vi "Error Code Dialog.vi"(8 "error in":errorcluster, 10 "Library":refnum<class "Library.lvclass">, 11 "Project":refnum<class "Project.lvclass">) -> (0 "error out":errorcluster, 1 "Cancel Out":bool, 2 "Error Name":string, 3 "Project out":refnum<class "Project.lvclass">, 5 "Error VI Tag":string)   [LabVIEW 2020, in "Panther Dashboard.lvlib"]
uses:
  Panther Dashboard.lvlib
  Controls/Continue.ctl
  Controls/Cancel.ctl
  Controls/MulticolumListbox.ctl
  Class/Library/Library.lvclass
  C:/GitClones/PantherDashboard/src/LabVIEW/Panther Dashboard/Class/LabVIEWItem/LabVIEWItem.lvclass
  Class/Project/Project.lvclass
  Class/Project/Project.lvclass/Project.ctl
  Class/Library/Library.lvclass/Library.ctl
  Class/LabVIEWItem/LabVIEWItem.lvclass/LabVIEWItem.ctl
  Class/LabVIEWItem/Item Type--enum.ctl
  Class/LabVIEWItem/Read Item Tag.vi
  Class/Project/Read Project Ref.vi
  Class/Project/Read Main App Inst Ref.vi
  Class/Library/Read Library Ref.vi
  Class/Library/Read Type.vi
  Class/VI/VI.lvclass
  Class/LabVIEWItem/LabVIEWItem.lvclass
panel:
  in  "Error Description":string
  in  "Current Error VIs Values":T1
  in  "Error Name (do not add --error.vi)":string
  in  "Continue":T2
  in  "Cancel":T3
  in  "Error Code":i32
  # "These are the benefits of having Error Constant VIs\n\n1. Centralized Error Management:\n   - Single Point of Editing: by storing error codes and descriptions in constants, you can modify them in one place, ensuring consistency across the entire application. This streamlines maintenance and avoids potential errors due to inconsistencies.\n   - Enhanced Organization: Grouping error-related information in constants improves code readability and understanding. It also makes it easier to quickly locate and update error-related logic.\n\n2. Improved Code Readability:\n   - Clearer Meaning: Instead of using raw error codes directly in code, constants provide meaningful names for errors, making code more self-explanatory and easier for others to comprehend.\n   - Reduced Redundancy: Constants eliminate the need to repeatedly define error codes and descriptions throughout the code, reducing redundancy and improving code maintainability.\n\n3. Error Tracking and Debugging:\n   - Identifying Error Sources: By using constant VIs, you can easily track where specific errors are being generated within the application. This aids in debugging and pinpointing the root causes of issues.\n   - Debugging Efficiency: Constants make it easier to search for error-related code and analyze error handling logic, facilitating debugging and problem resolution.\n\n4. Flexibility for Customization:\n   - Adaptability: If error codes or descriptions need to change, you can easily update them in the constant VIs without having to modify code in multiple locations. This allows for quick adjustments and customization as needed.\n\nRanges of Custom Error Codes defined by NI:\n     –8999  through –8000\n       5000  through   9999\n  500,000  through 599,999"
  # "TIP: Doble click to open --error.vi Block Diagram"
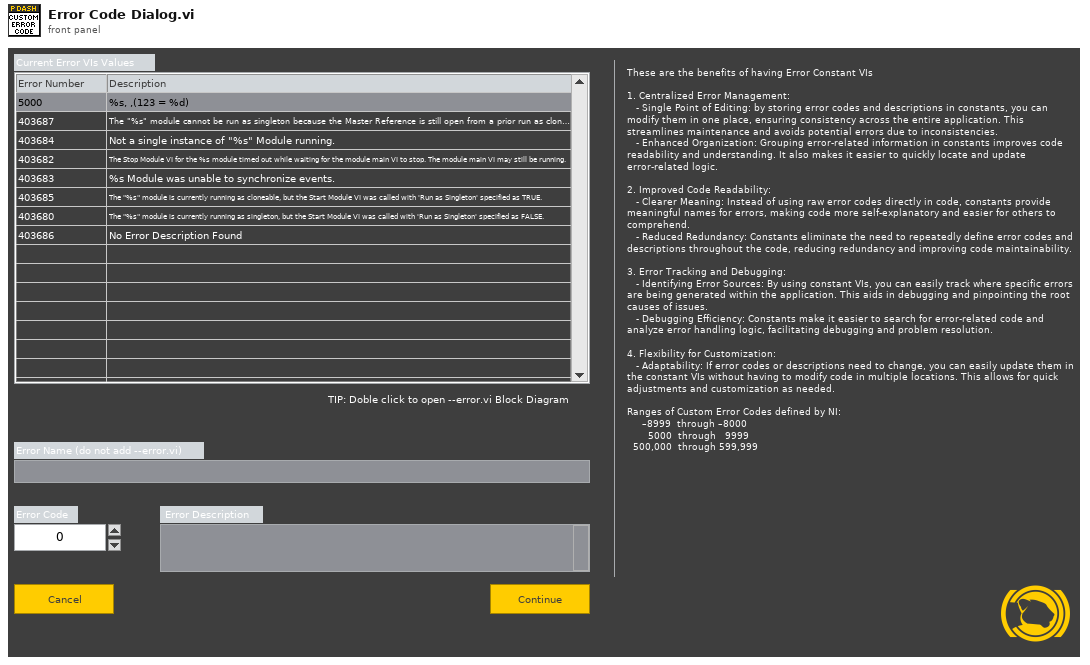
[diagram p1: front panel]
types:
  T1 = typedef "MulticolumListbox.ctl" = i32
  T2 = typedef "Continue.ctl" = bool
  T3 = typedef "Cancel.ctl" = bool
  T4 = typedef "Panther Dashboard.lvlib/Module type--enum.ctl" = enum16{"Singleton", "Cloneable"}
  T5 = typedef "Panther Dashboard.lvlib/LabVIEWItem.lvclass/Item Type--enum.ctl" = enum16{"Requests", "Broadcasts", "Request and Wait for Reply", "Round Trip", "» Public API VIs", "» Constant VIs", "» Error VIs", "Module", "Project", "No Drag Selection"}
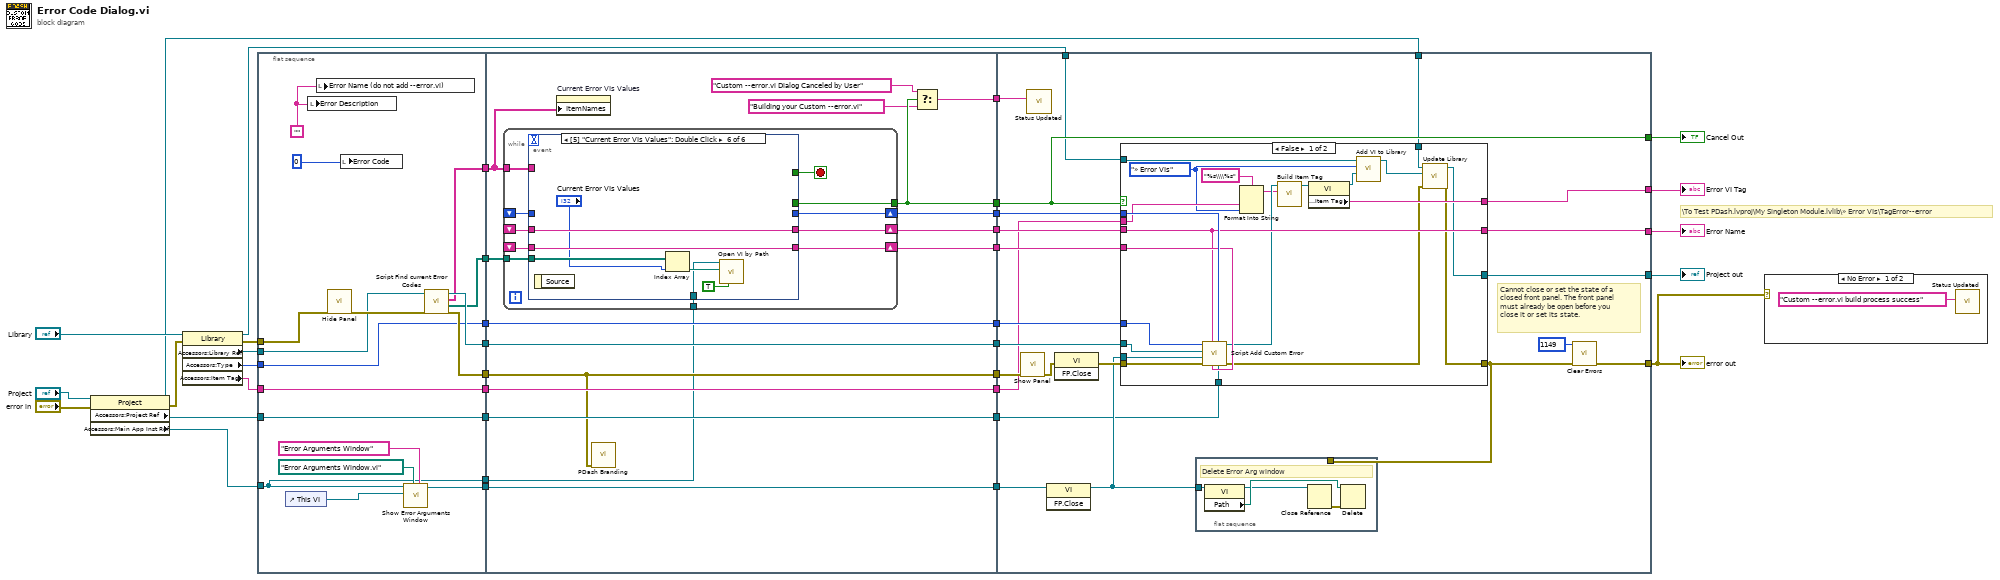
[diagram p0: block diagram]
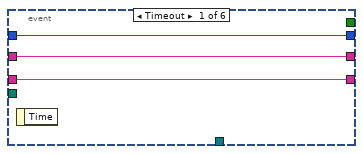
[diagram p3: hidden frame]
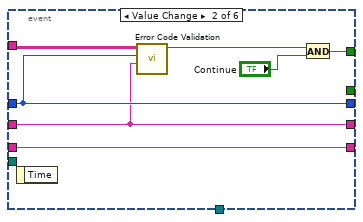
[diagram p4: hidden frame]
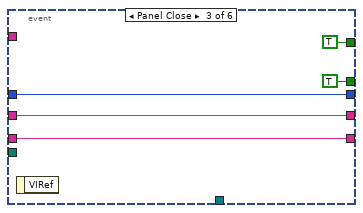
[diagram p5: hidden frame]
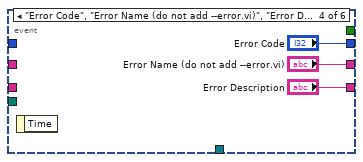
[diagram p6: hidden frame]
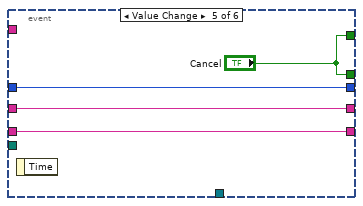
[diagram p7: hidden frame]
diagram:
  # "\\To Test PDash.lvproj\\My Singleton Module.lvlib\\» Error VIs\\TagError--error"
  n1 = property class="Project"(reference="Project", error in="error in") -> (reference out=w5:refnum<class "Project.lvclass">, error out=w33:errorcluster, "Accessors:Project Ref"=w15:refnum<vi>, "Accessors:Main App Inst Ref"=w14:refnum<vi>)
  n2 = property class="Library"(reference="Library", error in=w33) -> (reference out=w10:refnum<class "Library.lvclass">, error out=w35:errorcluster, "Accessors:Library Ref"=w12:refnum<vi>, "Accessors:Type"=w11:T4, "Accessors:Item Tag"=w8:string)
  n3 = flat-sequence {
    tunnel: w12 -> [w50]
    tunnel: w35 -> [w54]
    tunnel: [w53] -> w37
    tunnel: [w49] -> w28
    tunnel: [w48] -> w27
    tunnel: [w46] -> w25
    tunnel: w14 -> [w38]
    tunnel: w11 -> [w45]
    tunnel: [w45] -> w24
    tunnel: [w41] -> w19
    tunnel: w15 -> [w41]
    tunnel: [w40] -> w9
    tunnel: w8 -> [w40]
    tunnel: [w39] -> w2
    tunnel: [w38] -> w1
    tunnel: w37 -> [w59]
    tunnel: [w59] -> w36
    tunnel: [w65] -> w32
    tunnel: [w70] -> w31
    tunnel: [w69] -> w30
    tunnel: [w68] -> w29
    tunnel: w28 -> [w68]
    tunnel: w27 -> [w58]
    tunnel: [w56] -> w26
    tunnel: w25 -> [w56]
    tunnel: w24 -> [w67]
    tunnel: [w67] -> w23
    tunnel: [w66] -> w22
    tunnel: [w62] -> w21
    tunnel: [w61] -> w20
    tunnel: w19 -> [w61]
    tunnel: w9 -> [w60]
    tunnel: [w60] -> w7
    tunnel: w2 -> [w57]
    tunnel: w1 -> [w55]
    tunnel: [w132] -> w3
    tunnel: w36 -> [w129]
    tunnel: w32 -> [w116]
    tunnel: w31 -> [w127]
    tunnel: w30 -> [w126]
    tunnel: w29 -> [w125]
    tunnel: w26 -> [w122]
    tunnel: w23 -> [w124]
    tunnel: w22 -> [w120]
    tunnel: w21 -> [w119]
    tunnel: w20 -> [w118]
    tunnel: [w117] -> w18
    tunnel: [w116] -> w17
    tunnel: w10 -> [w115]
    tunnel: w7 -> [w114]
    tunnel: [w113] -> w6
    tunnel: w5 -> [w112]
    tunnel: [w111] -> w4
    frame #0 {
      w42 = "" ("Error Message")
      n4 = control-ref of="This VI"() -> (w47:refnum<vi>)
      n5 = local write "Error Description"(w42) -> ()
      n6 = local write "Error Name (do not add --error.vi)"(w42) -> ()
      n7 = call "Hide Panel.vi"("error in (no error)"=w54) -> ("error out"=w52:errorcluster)  [unwired: 10 in]
      n8 = local write "Error Code"(0 ("Error Code")) -> ()
      n9 = call "Show Error Arguments Window.vi"("Title"="Error Arguments Window", "Path"=path "Error Arguments Window.vi", "Calling VI Ref"=w47, "App Instance"=w38) -> ("Error Arguments Window Ref"=w46:refnum<vi>)  [unwired: 6 in, 1 out]
      n10 = call "Script Find current Error Codes.vi"("error in"=w52, "Library in"=w50) -> ("error out"=w53:errorcluster, "All Error VIS"=w39:path[], "Error and Descriptions Table"=w48:string[][], "Library out"=w49:refnum<vi>)  [unwired: 6 in]
    }
    frame #1 {
      n11 = while {
        shift-right: [w80] -> w69
        shift-left: _ -> [w79]
        shift-right: [w78] -> w70
        shift-left: _ -> [w77]
        tunnel: [w76] -> w65
        tunnel: w58 -> [w75]
        shift-right: [w74] -> w66
        shift-left: _ -> [w73]
        tunnel: w57 -> [w72]
        tunnel: w55 -> [w71]
        stop <- w81 stop-if-true
        n12 = event shown="[5] \"Current Error VIs Values\": Double Click" {
          selector: _ -> [_ _ _ _ _ _]
          dyn-events: _ -> [_ _ _ _ _ _]
          timeout: _ -> [_ _ _ _ _ _]
          tunnel: [_ w90 TRUE ("Cancel") _ "Cancel" _] -> w81
          tunnel: [w84 w91 w92 "Error Code" w102 _] -> w80
          tunnel: w79 -> [w84 w91 w92 _ w102 _]
          tunnel: [w83 w85 w96 "Error Name (do not add --error.vi)" w103 w110] -> w78
          tunnel: w77 -> [w83 w85 w96 _ w103 w110]
          tunnel: [_ _ TRUE ("Cancel") _ "Cancel" _] -> w76
          tunnel: w75 -> [_ w87 _ _ _ _]
          tunnel: [w82 w86 w93 "Error Description" w100 w109] -> w74
          tunnel: w73 -> [w82 w86 w93 _ w100 w109]
          tunnel: w72 -> [_ _ _ _ _ w108]
          tunnel: w71 -> [_ _ _ _ _ w105]
          event Timeout {
            n13 = event-data() -> ()  [unwired: 1 in, 1 out]
          }
          event Value Change {
            n14 = event-data() -> ()  [unwired: 1 in, 1 out]
            n15 = call "Error Code Validation.vi"("Error Name"=w85, "New Error Code"=w91, "Error Codes and Descriptions"=w87) -> ("Continue"=w88:bool)  [unwired: 8 in]
            n16 = And(x=w88, y="Continue") -> (x .and. y?=w90:T2)
          }
          event Panel Close {
            n17 = event-data() -> ()  [unwired: 1 in, 1 out]
          }
          event "Error Code", "Error Name (do not add --error.vi)", "Error Description": Value Change {
            n18 = event-data() -> ()  [unwired: 1 in, 1 out]
          }
          event Value Change {
            n19 = event-data() -> ()  [unwired: 1 in, 1 out]
          }
          event Double Click {
            n20 = event-data() -> ()  [unwired: 1 in, 1 out]
            n21 = Index Array(array=w108, index="Current Error VIs Values") -> (element=w106:path)
            n22 = call "Open VI by Path.vi"("Block Diagram?"=TRUE, "VI Path"=w106, "Application in"=w105) -> ()  [unwired: 8 in, 1 out]
          }
        }
      }
      n23 = property on="Current Error VIs Values" class="MCListbox (strict)"("ItemNames"=w58) -> ()  [unwired: 2 in, 2 out]
      n24 = call "PDash Branding.vi"("error in"=w59) -> ()  [unwired: 11 in]
      n25 = Select(t="Custom --error.vi Dialog Canceled by User" ("Status"), s=w65, f="Building your Custom --error.vi" ("Status")) -> (s? t:f=w62:string)
    }
    frame #2 {
      # "Cannot close or set the state of a closed front panel. The front panel must already be open before you close it or set its state."
      n26 = call "Show Panel.vi"("error in (no error)"=w129) -> ("error out"=w128:errorcluster)  [unwired: 10 in]
      n27 = call "Status Updated.vi"("Status"=w119) -> ()  [unwired: 10 in, 1 out]
      n28 = invoke class="VI" method="FP.Close"(reference=w122) -> (reference out=w121:refnum<vi>)  [unwired: 2 in, 2 out]
      n29 = invoke class="VI" method="FP.Close"(error in=w128) -> (error out=w131:errorcluster)  [unwired: 2 in, 2 out]
      n30 = case shown="False" w116 {
        tunnel: [w137 w161] -> w130
        tunnel: w131 -> [w158 w161]
        tunnel: w127 -> [w151 w160]
        tunnel: w126 -> [w157 _]
        tunnel: w125 -> [w156 _]
        tunnel: w121 -> [w155 _]
        tunnel: w124 -> [w154 _]
        tunnel: w120 -> [w153 _]
        tunnel: w118 -> [w152 _]
        tunnel: [w151 w160] -> w117
        tunnel: w115 -> [w150 _]
        tunnel: w114 -> [w145 _]
        tunnel: [w146 _] -> w113
        tunnel: w112 -> [w140 w159]
        tunnel: [w139 w159] -> w111
        frame False {
          w144 = Item_Type--enum."» Error VIs" ("VI Type")
          n31 = call "Script Add Custom Error.vi"("Project Reference"=w152, "Error Code"=w157, "Error Description"=w153, "Error Name"=w151, "error in"=w158, "Error Arguments Window Ref"=w155, "DQMH Lib Ref"=w156, "Module type"=w154) -> ("error out"=w138:errorcluster, "VI out"=w149:refnum<class "VI.lvclass">)  [unwired: 2 in]
          n32 = Format Into String(format string="%s\\\\%s", w145, w144) -> (resulting string=w143:string)  [unwired: 2 in, 1 out]
          n33 = call "Build Item Tag.vi"("Parent Tag"=w143, "LabVIEWItem in"=w149) -> ("LabVIEWItem out"=w148:refnum<class "VI.lvclass">)  [unwired: 8 in, 1 out]
          n34 = property class="VI"(reference=w148) -> (reference out=w147:refnum<class "VI.lvclass">, "Accessors:Item Tag"=w146:string)  [unwired: 1 in, 1 out]
          n35 = call "Add VI to Library.vi"("VI"=w147, "VI Type"=w144, "Library in"=w150) -> ("Library out"=w141:refnum<class "Library.lvclass">)  [unwired: 7 in, 1 out]
          n36 = call "Update Library.vi"("error in"=w138, "Library"=w141, "Project in"=w140) -> ("error out"=w137:errorcluster, "Project out"=w139:refnum<class "Project.lvclass">)  [unwired: 7 in]
        }
        frame True {
        }
      }
      n37 = flat-sequence {
        tunnel: w121 -> [w135]
        tunnel: w130 -> [_]
        frame #0 {
          # "Delete Error Arg window"
          n38 = property class="VI"(reference=w135) -> (reference out=w133:refnum<vi>, "Path"=w134:path)  [unwired: 1 in, 1 out]
          n39 = Close Reference(reference=w133) -> (error out=w136:errorcluster)  [unwired: 1 in]
          n40 = Delete(path (use dialog)=w134, error in=w136) -> ()  [unwired: 3 in, 3 out]
        }
      }
      n41 = call <vilib>:"Clear Errors.vi"("error in (no error)"=w130, "specific error code to clear (0: all)"=1149) -> ("error out"=w132:errorcluster)  [unwired: 4 in, 1 out]
    }
  }
  n42 = case shown="No Error" w3 {
    frame No Error {
      n43 = call "Status Updated.vi"("Status"="Custom --error.vi build process success") -> ()  [unwired: 10 in, 1 out]
    }
    frame Error {
    }
  }
  "error out" <- w3
  "Error Name" <- w18
  "Cancel Out" <- w17
  "Project out" <- w4
  "Error VI Tag" <- w6
